vi "System Monitor RT Driver VI.vi"(6 "Device Clock":string, 9 "Device Inputs FIFO":refnum<k33>, 10 "Device Outputs FIFO":refnum<k33>, 11 "Device Reference":T1 format="%.0x") -> ()   [LabVIEW 2011, in "System Monitor Custom Device.lvlib"]
uses:
  System Monitor Custom Device.lvlib
  <vilib>/NI Veristand/Custom Device API/Custom Device Channel Type.ctl
  <vilib>/NI Veristand/Custom Device API/Custom Device API.lvlib
  <vilib>/NI Veristand/Custom Device Tools/Custom Device Utility Library/Custom Device Utility Library.lvlib
  <vilib>/NI Veristand/Custom Device API/Get Item Property (I32).vi
  <vilib>/NI Veristand/Custom Device API/Custom Device Item Ref.ctl
panel:
  in  "Status Notifier":refnum<notifier>
  # "Custom Device Template\nv1.0"
  # "Use this template as a starting point for creating a custom device code module. The input controls shown here are specially named controls that the system will use to provide the device loop with data. The controls are not required for the device loop to run. For instance, if the device doesn't produce any output data, then you don't need the Device Outputs FIFO control. If you do use these controls, however, they need to have these exact names to be functional."
  # "The optional status notifier element is used to notify the RT engine of the last state of the custom device, and to indicate the device has completed execution. If this control is not used, a default No Error value is returned to the system when the device finishes execution.\n\nNote: This error state is not checked until the system shuts down. Use an output status channel to send more immediate status values to the system."
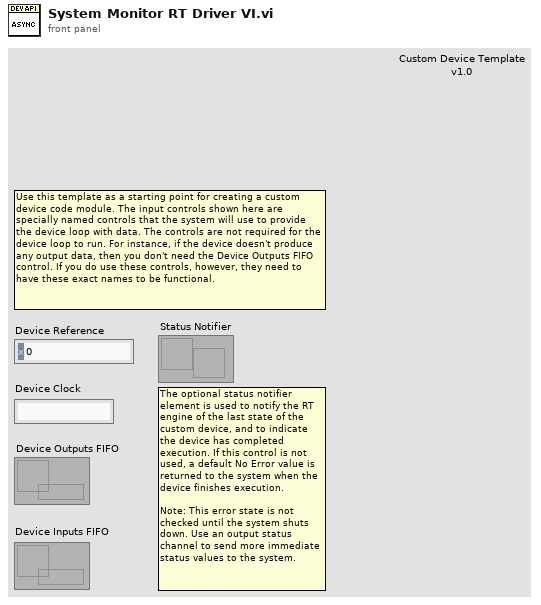
[diagram p1: front panel]
types:
  T1 = typedef "Custom Device API.lvlib/Custom Device Item Ref.ctl" = u64
  T2 = typedef "Custom Device API.lvlib/Custom Device Channel Type.ctl" = enum16{"Input", "Output"}
  T3 = typedef "NI_Real-Time Target Support.lvlib/RT CPU Load.ctl" = cluster{"Total (%)":dbl, "Time Critical (%)":dbl, "Timed Structures (%)":dbl, "High (%)":dbl, "Above Normal (%)":dbl, "Normal (%)":dbl, "Background (%)":dbl, "Idle (%)":dbl, "ISR (%)":dbl}
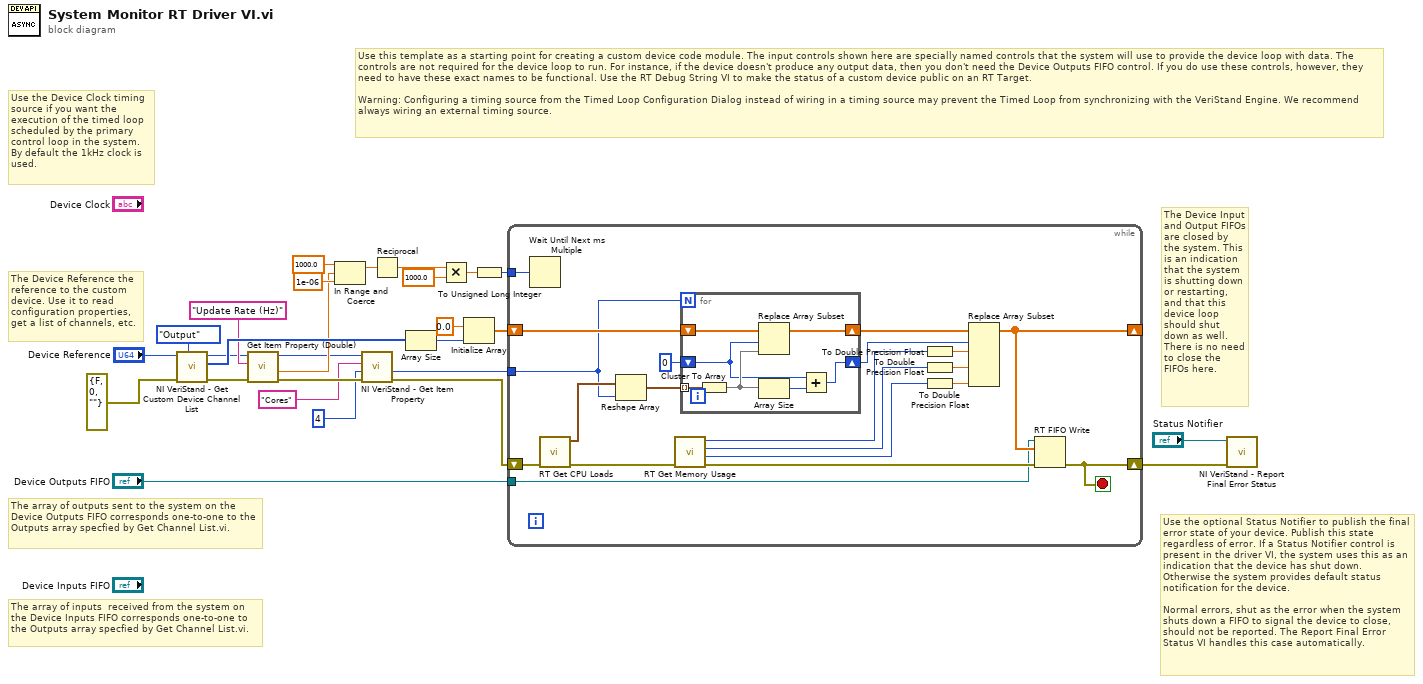
[diagram p0: block diagram]
diagram:
  # "The array of inputs  received from the system on the Device Inputs FIFO corresponds one-to-one to the Outputs array specfied by Get Channel List.vi."
  # "Use the optional Status Notifier to publish the final error state of your device. Publish this state regardless of error. If a Status Notifier control is present in the driver VI, the system uses this as an indication that the device has shut down. Otherwise the system provides default status notification for the device.\n\nNormal errors, shut as the error when the system shuts down a FIFO to signal the device to close, should not be reported. The Report Final Error Status VI handles this case automatically."
  # "The Device Input and Output FIFOs are closed by the system. This is an indication that the system is shutting down or restarting, and that this device loop should shut down as well. There is no need to close the FIFOs here."
  # "The array of outputs sent to the system on the Device Outputs FIFO corresponds one-to-one to the Outputs array specfied by Get Channel List.vi."
  # "The Device Reference the reference to the custom device. Use it to read configuration properties, get a list of channels, etc."
  # "Use the Device Clock timing source if you want the execution of the timed loop scheduled by the primary control loop in the system. \nBy default the 1kHz clock is used."
  # "Use this template as a starting point for creating a custom device code module. The input controls shown here are specially named controls that the system will use to provide the device loop with data. The controls are not required for the device loop to run. For instance, if the device doesn't produce any output data, then you don't need the Device Outputs FIFO control. If you do use these controls, however, they need to have these exact names to be functional. Use the RT Debug String VI to make the status of a custom device public on an RT Target.\n\nWarning: Configuring a timing source from the Timed Loop Configuration Dialog instead of wiring in a timing source may prevent the Timed Loop from synchronizing with the VeriStand Engine. We recommend always wiring an external timing source."
  n1 = call <vilib>:"NI VeriStand - Get Custom Device Channel List.vi"("Channel Type"=Custom_Device_Channel_Type."Output", "error in (no error)"=errorcluster {"status"=FALSE, "code"=0, "source"=""}, "Device Ref in"="Device Reference") -> ("error out"=w9:errorcluster, "Specified Channel Ref List"=w24:T1[], "Device Ref out"=w10:T1)  [unwired: 6 out]
  n2 = call <vilib>:"Get Item Property (Double).vi"("error in (no error)"=w9, "Property Name"="Update Rate (Hz)", "Item Ref in"=w10) -> ("error out"=w5:errorcluster, "Value"=w8:dbl, "Item Ref out"=w6:T1)  [unwired: 5 in, 1 out]
  n3 = In Range and Coerce(upper limit=1000.0, x=w8, lower limit=1e-06 ("x")) -> (coerced(x)=w16:dbl)  [unwired: 1 out]
  n4 = call-poly <vilib>:"NI VeriStand - Get Item Property.vi"("error in (no error)"=w5, "Default Value"=4, "Property Name"="Cores", "Item Ref in"=w6) -> ("error out"=w2:errorcluster, "Value"=w1:i32)  [unwired: 4 in, 2 out]
  n5 = Reciprocal(x=w16) -> (1/x=w13:dbl)
  n6 = Array Size(array=w24) -> (size(s)=w25:i32)
  n7 = Multiply(x=w13, y=1000.0) -> (x*y=w15:dbl)
  n8 = Initialize Array(0.0 ("element"), w25) -> (w22:dbl[])
  n9 = To Unsigned Long Integer(number=w15) -> (unsigned 32bit integer=w12:u32)
  n10 = while {
    shift-right: [w31] -> _
    shift-left: w22 -> [w45]
    shift-right: [w32] -> w7
    shift-left: w2 -> [w47]
    tunnel: "Device Outputs FIFO" -> [w30]
    tunnel: w12 -> [w29]
    tunnel: w1 -> [w28]
    stop <- w32 stop-if-true
    n11 = Wait Until Next ms Multiple(millisecond multiple=w29) -> ()  [unwired: 1 out]
    n12 = call <vilib>:"RT Get CPU Loads.vi"("error in (no error)"=w47) -> ("error out"=w46:errorcluster, "CPU loads"=w34:T3[])  [unwired: 9 in]
    n13 = Reshape Array(w34, w28) -> (w35:T3[])
    n14 = call <vilib>:"RT Get Memory Usage.vi"("error in (no error)"=w46) -> ("error out"=w33:errorcluster, "largest contiguous (bytes)"=w36:u32, "available (bytes)"=w37:u32, "total (bytes)"=w41:u32)  [unwired: 7 in]
    n15 = for {
      N: w28 -> [_]
      tunnel: w35 -> [w48] mode=indexing
      shift-right: [w53] -> w43
      shift-left: w45 -> [w54]
      shift-right: [w51] -> w42
      shift-left: 0 -> [w49]
      n16 = Cluster To Array(cluster=w48) -> (array=w50:dbl[])
      n17 = Replace Array Subset(array=w54, new element=w50, index=w49) -> (w53:dbl[])
      n18 = Array Size(array=w50) -> (size(s)=w52:i32)
      n19 = Add(x=w49, y=w52) -> (x+y=w51:i32)
    }
    n20 = To Double Precision Float(number=w41) -> (double precision float=w40:dbl)
    n21 = To Double Precision Float(number=w37) -> (double precision float=w39:dbl)
    n22 = To Double Precision Float(number=w36) -> (double precision float=w38:dbl)
    n23 = Replace Array Subset(array=w43, new element #1=w40, index #1=w42, new element #2=w39, new element #3=w38) -> (w31:dbl[])  [unwired: 2 in]
    n24 = RT FIFO Write(0:w30, 1:w31, 3:w33) -> (11:w32:errorcluster)  [unwired: 2 in, 3 out]
  }
  n25 = call <vilib>:"NI VeriStand - Report Final Error Status.vi"("error in (no error)"=w7, "Status Notifier"="Status Notifier") -> ()  [unwired: 1 in, 9 out]
